vi "2021 Advent puzzle 05 Add via lines.vi"(6 "Y2":i32[](array[numeric]), 7 "Allow diag":bool, 8 "X2":i32[](array[numeric]), 9 "Y1":i32[](array[numeric]), 10 "X1":i32[](array[numeric]), 11 "Array in":i16[][](array[numeric])) -> (3 "Array out":i16[][](array[numeric]))   [LabVIEW 2021]
panel:
  out "Array out 4":i16[][](array[numeric])
  out "Loop":i32
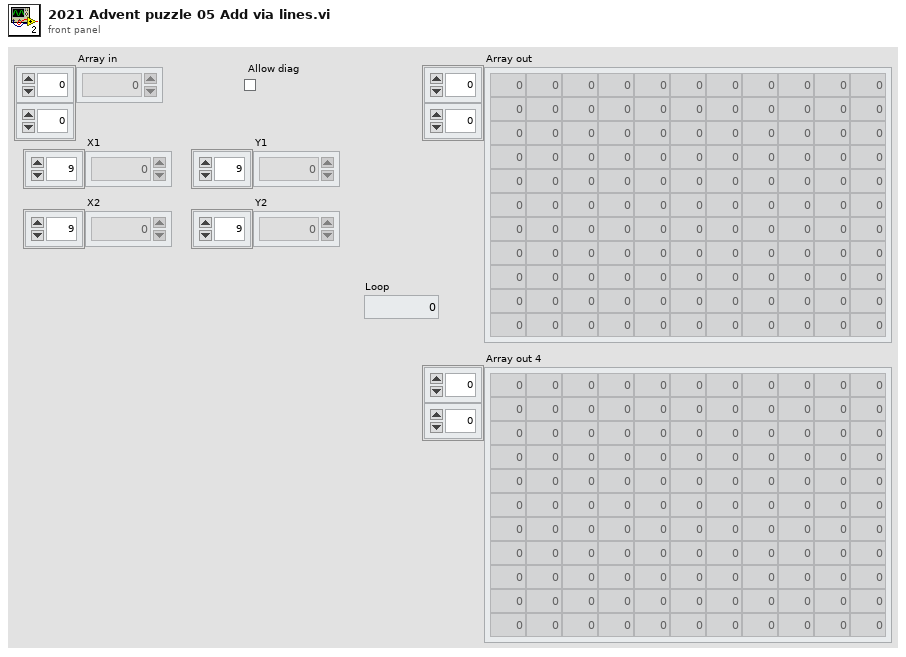
[diagram p1: front panel]
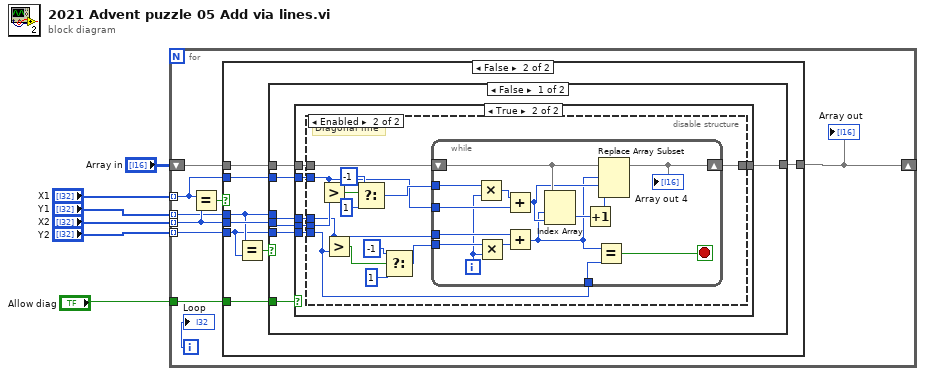
[diagram p0: block diagram]
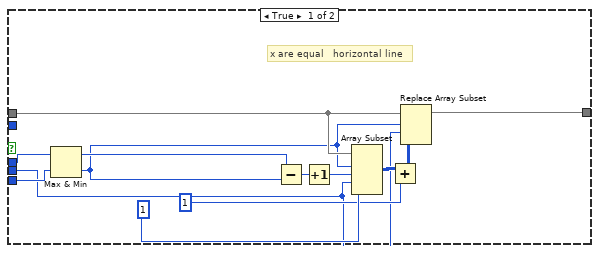
[diagram p2: hidden frame]
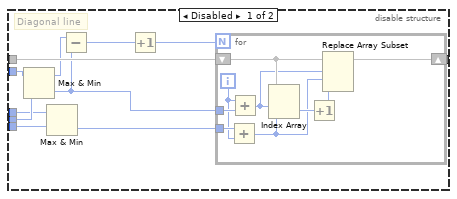
[diagram p4: hidden frame]
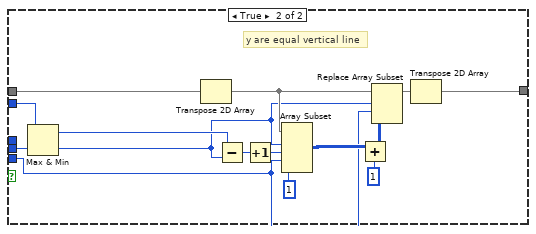
[diagram p5: hidden frame]
diagram:
  n1 = for {
    tunnel: "X1" -> [w12] mode=indexing
    tunnel: "X2" -> [w14] mode=indexing
    tunnel: "Y1" -> [w13] mode=indexing
    tunnel: "Y2" -> [w11] mode=indexing
    shift-right: [w8] -> _
    shift-left: "Array in" -> [w10]
    tunnel: "Allow diag" -> [w9]
    i -> [w7]
    n2 = Equal?(x=w12, y=w14) -> (x = y?=w15:bool)
    n3 = case shown="False" w15 {
      tunnel: w14 -> [w17 w35]
      tunnel: w13 -> [w19 w32]
      tunnel: w12 -> [_ w30]
      tunnel: w11 -> [w18 w31]
      tunnel: w10 -> [w28 w36]
      tunnel: [w20 w34] -> w8
      tunnel: w9 -> [_ w29]
      frame True {
        # "x are equal   horizontal line"
        n4 = Max & Min(x=w19, y=w18) -> (max(x,y)=w27:i32, min(x,y)=w21:i32)
        n5 = Subtract(x=w27, y=w21) -> (x-y=w26:i32)
        n6 = Increment(x=w26) -> (x+1=w16:i32)
        n7 = Array Subset(array=w28, index (row)=w21, length (row)=w16, index (col)=w17, length (col)=1 ("length")) -> (w25:i16[][])
        n8 = Add(x=w25, y=i16 1) -> (x+y=w22:i16[][])
        n9 = Replace Array Subset(array=w28, new element=w22, index (row)=w21, index (col)=w17) -> (w20:i16[][])
      }
      frame False {
        n10 = Equal?(x=w32, y=w31) -> (x = y?=w33:bool)
        n11 = case shown="False" w33 {
          tunnel: w36 -> [w43 w114]
          tunnel: w32 -> [w37 _]
          tunnel: w31 -> [w38 w101]
          tunnel: w35 -> [w39 w102]
          tunnel: [w42 w104] -> w34
          tunnel: w30 -> [w40 w103]
          tunnel: w29 -> [w41 _]
          frame False {
            n12 = case shown="True" w41 {
              tunnel: w43 -> [w44 w46]
              tunnel: [w44 w45] -> w42
              tunnel: w40 -> [_ w50]
              tunnel: w39 -> [_ w49]
              tunnel: w38 -> [_ w48]
              tunnel: w37 -> [_ w47]
              frame False {
              }
              frame True {
                n13 = disable-structure shown="Enabled" {
                  disable-tunnel: w50 -> [w61 w72]
                  disable-tunnel: w49 -> [w60 w82]
                  disable-tunnel: w48 -> [w59 w71]
                  disable-tunnel: w47 -> [w58 w73]
                  disable-tunnel: w46 -> [w57 w84]
                  disable-tunnel: [w56 w83] -> w45
                  frame Disabled {
                    # "Diagonal line"
                    n14 = Max & Min(x=w61, y=w60) -> (max(x,y)=w55:i32, min(x,y)=w52:i32)
                    n15 = Max & Min(x=w58, y=w59) -> (min(x,y)=w51:i32)  [unwired: 1 out]
                    n16 = Subtract(x=w55, y=w52) -> (x-y=w54:i32)
                    n17 = Increment(x=w54) -> (x+1=w53:i32)
                    n18 = for {
                      N: w53 -> [_]
                      shift-right: [w69] -> w56
                      shift-left: w57 -> [w70]
                      tunnel: w52 -> [w66]
                      tunnel: w51 -> [w67]
                      i -> [w63]
                      n19 = Add(x=w67, y=w63) -> (x+y=w64:i32)
                      n20 = Add(x=w63, y=w66) -> (x+y=w65:i32)
                      n21 = Index Array(array=w70, index (row)=w65, index (col)=w64) -> (element=w68:i16)
                      n22 = Increment(x=w68) -> (x+1=w62:i16)
                      n23 = Replace Array Subset(array=w70, new element=w62, index (row)=w65, index (col)=w64) -> (w69:i16[][])
                    }
                  }
                  frame Enabled {
                    # "Diagonal line"
                    n24 = Greater?(x=w72, y=w82) -> (0:w81:bool)
                    n25 = Greater?(x=w73, y=w71) -> (0:w74:bool)
                    n26 = Select(t=-1, s=w81, f=1) -> (s? t:f=w78:i32)
                    n27 = Select(t=-1, s=w74, f=1) -> (s? t:f=w75:i32)
                    n28 = while {
                      shift-right: [w98] -> w83
                      shift-left: w84 -> [w99]
                      tunnel: w72 -> [w95]
                      tunnel: w73 -> [w96]
                      tunnel: w71 -> [w93]
                      tunnel: w78 -> [w91]
                      tunnel: w75 -> [w90]
                      i -> [w87]
                      stop <- w92 stop-if-true
                      n29 = Multiply(x=w91, y=w87) -> (x*y=w88:i32)
                      n30 = Multiply(x=w90, y=w87) -> (x*y=w89:i32)
                      n31 = Add(x=w88, y=w95) -> (x+y=w86:i32)
                      n32 = Add(x=w96, y=w89) -> (x+y=w85:i32)
                      n33 = Index Array(array=w99, index (row)=w85, index (col)=w86) -> (element=w97:i16)
                      n34 = Increment(x=w97) -> (x+1=w94:i16)
                      n35 = Equal?(x=w85, y=w93) -> (x = y?=w92:bool)
                      n36 = Replace Array Subset(array=w99, new element=w94, index (row)=w85, index (col)=w86) -> (w98:i16[][])
                      "Array out 4" <- w98
                    }
                  }
                }
              }
            }
          }
          frame True {
            # "y are equal vertical line"
            n37 = Max & Min(x=w103, y=w102) -> (max(x,y)=w113:i32, min(x,y)=w106:i32)
            n38 = Transpose 2D Array(2D array=w114) -> (transposed array=w108:i16[][])
            n39 = Subtract(x=w113, y=w106) -> (x-y=w112:i32)
            n40 = Increment(x=w112) -> (x+1=w100:i32)
            n41 = Array Subset(array=w108, index (row)=w106, length (row)=w100, index (col)=w101, length (col)=1 ("length")) -> (w111:i16[][])
            n42 = Add(x=w111, y=i16 1) -> (x+y=w107:i16[][])
            n43 = Replace Array Subset(array=w108, new element=w107, index (row)=w106, index (col)=w101) -> (w105:i16[][])
            n44 = Transpose 2D Array(2D array=w105) -> (transposed array=w104:i16[][])
          }
        }
      }
    }
    "Array out" <- w8
    "Loop" <- w7
  }
